vi "Q2_validar torre.vi"(2 "coordenadas del mouse":T1) -> (4 "Torre":i32, 5 "torre1":bool, 6 "torre2":bool, 7 "torre3":bool)   [LabVIEW 2020]
uses:
  <vilib>/Utility/miscctls.llb/LVPoint32TypeDef.ctl
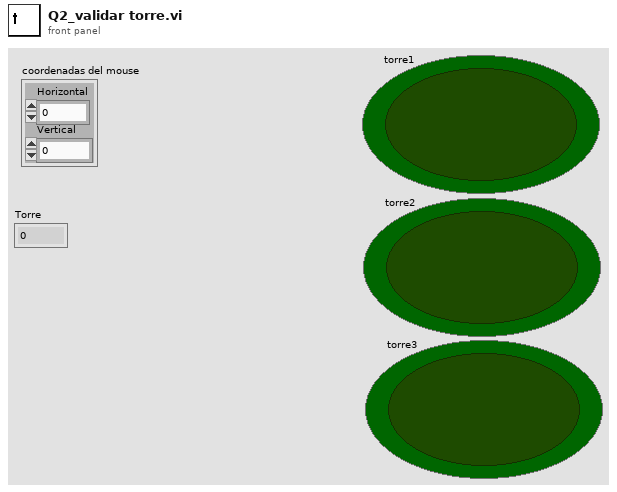
[diagram p1: front panel]
types:
  T1 = typedef "LVPoint32TypeDef.ctl" = cluster{"Horizontal":i32, "Vertical":i32}
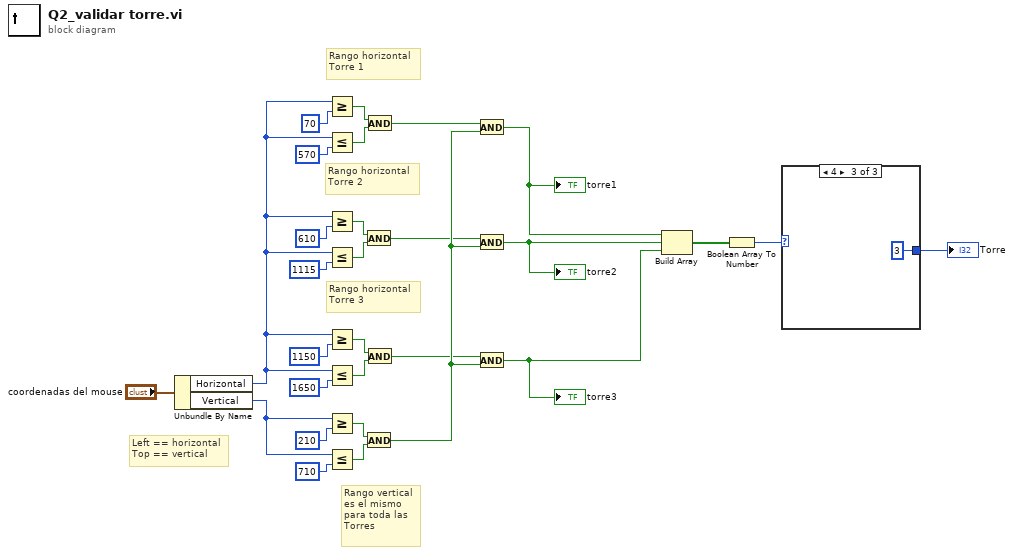
[diagram p0: block diagram]
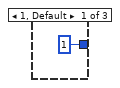
[diagram p2: hidden frame]
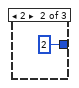
[diagram p3: hidden frame]
diagram:
  # "Rango horizontal\nTorre 3"
  # "Rango horizontal\nTorre 2"
  # "Rango horizontal\nTorre 1"
  # "Rango vertical\nes el mismo \npara toda las\nTorres"
  # "Left == horizontal\nTop == vertical"
  n1 = Unbundle By Name("coordenadas del mouse") -> ("Horizontal"=w28:i32, "Vertical"=w29:i32)
  n2 = Greater Or Equal?(x=w28, y=70 ("Vertical")) -> (x >= y?=w11:bool)
  n3 = Less Or Equal?(x=w28, y=570 ("Vertical")) -> (x <= y?=w10:bool)
  n4 = Greater Or Equal?(x=w28, y=610 ("Vertical")) -> (x >= y?=w16:bool)
  n5 = Less Or Equal?(x=w28, y=1115 ("Vertical")) -> (x <= y?=w17:bool)
  n6 = Greater Or Equal?(x=w28, y=1150 ("Vertical")) -> (x >= y?=w23:bool)
  n7 = Less Or Equal?(x=w28, y=1650 ("Vertical")) -> (x <= y?=w22:bool)
  n8 = Greater Or Equal?(x=w29, y=210 ("Vertical")) -> (x >= y?=w12:bool)
  n9 = Less Or Equal?(x=w29, y=710 ("Vertical")) -> (x <= y?=w13:bool)
  n10 = And(x=w16, y=w17) -> (x .and. y?=w25:bool)
  n11 = And(x=w12, y=w13) -> (x .and. y?=w27:bool)
  n12 = And(x=w11, y=w10) -> (x .and. y?=w24:bool)
  n13 = And(x=w23, y=w22) -> (x .and. y?=w26:bool)
  n14 = And(x=w24, y=w27) -> (x .and. y?=w7:bool)
  "torre1" <- w7
  n15 = And(x=w25, y=w27) -> (x .and. y?=w2:bool)
  "torre2" <- w2
  n16 = And(x=w26, y=w27) -> (x .and. y?=w1:bool)
  "torre3" <- w1
  n17 = Build Array(w7, w2, w1) -> (w6:bool[])
  n18 = Boolean Array To Number(Boolean array=w6) -> (number=w5:u32)
  n19 = case shown="4" w5 {
    tunnel: [1 ("positionIncialTorre") 2 ("positionIncialTorre") 3 ("positionIncialTorre")] -> w3
    frame 1, Default {
    }
    frame 2 {
    }
    frame 4 {
    }
  }
  "Torre" <- w3
